vi "Lab Panel V5.26.vi"() -> ()   [LabVIEW 2017] (continued)
                          tunnel: w859 -> [_ _ w868]
                          tunnel: w858 -> [w866 w867 _]
                          tunnel: [w866 w867 w868] -> w857
                          frame "CHART TEST", Default {
                          }
                          frame "CYCLE TEST" {
                          }
                          frame "T-RISE TEST" {
                          }
                        }
                        n587 = local read "TDMS LAB01-2"() -> (w865:refnum<k34>)
                        n588 = Build Array("STOPPED") -> (w862:string[])
                        n589 = Build Array(w857) -> (w856:dbl[])
                        n590 = TDMS Write(0:w865, 5:"TEST RESULT", 7:w862, 9:w856) -> (4:w854:refnum<k34>, 15:w855:errorcluster)  [unwired: 2 in, 2 out]
                        n591 = TDMS Close(8:w855, 11:w854) -> (0:w853:errorcluster)  [unwired: 1 out]
                      }
                      frame #1 {
                        n592 = local read "DISP LAB01-2"() -> (w872:T4)
                        n593 = stacked-sequence {
                          tunnel: "LAB01-2" -> [w874 w876]
                          frame #0 {
                            n594 = call "sub vi - defrag tdms v1.vi"("panel id"=w874) -> ("error out"=w873:errorcluster)  [unwired: 10 in]
                            n595 = local write "data file error"(w873) -> ()
                          }
                          frame #1 {
                            n596 = call "Save data file (stop) v3.vi"("panel id"=w876) -> ("network file save error"=w875:errorcluster)  [unwired: 9 in, 1 out]
                            n597 = local write "RESULT LAB01-2"(FALSE) -> ()
                            n598 = local write "data file error"(w875) -> ()
                          }
                        }
                        n599 = Bundle(cluster=w872, "STATUS"="STOP") -> (w870:T4)  [unwired: 2 in]
                        n600 = local write "DISP LAB01-2"(w870) -> ()
                      }
                    }
                  }
                  frame True {
                    n601 = local read "SIG LAB01-2"() -> (w879:T2)
                    n602 = stacked-sequence {
                      seq-local: [w890 _] -> [_ w894]
                      tunnel: w888 -> [_ w904]
                      tunnel: w887 -> [_ w903]
                      tunnel: w886 -> [_ w902]
                      tunnel: w885 -> [_ w901]
                      tunnel: w884 -> [_ w900]
                      tunnel: [_ w899] -> w883
                      tunnel: w882 -> [_ w898]
                      tunnel: w881 -> [_ w897]
                      tunnel: w880 -> [_ w896]
                      tunnel: w879 -> [w889 w895]
                      tunnel: w878 -> [_ w893]
                      frame #0 {
                        n603 = Unbundle(w889) -> ("AMPS"=w892:dbl)  [unwired: 4 out]
                        n604 = call "Check For Amps on v1.vi"("ID"="LAB01-2", "amps"=w892) -> ("amps"=w890:bool)  [unwired: 9 in]
                      }
                      frame #1 {
                        n605 = case shown="True" w894 {
                          tunnel: w904 -> [_ w917]
                          tunnel: w903 -> [_ w916]
                          tunnel: w902 -> [_ w915]
                          tunnel: w901 -> [_ w914]
                          tunnel: w900 -> [_ w913]
                          tunnel: [errorcluster {"status"=FALSE, "code"=0, "source"=""} ("error out") w912] -> w899
                          tunnel: w898 -> [_ w911]
                          tunnel: w897 -> [_ w910]
                          tunnel: w896 -> [_ w909]
                          tunnel: w895 -> [_ w908]
                          tunnel: w893 -> [_ w907]
                          frame False {
                            w905 = FALSE
                            n606 = local write "RUN LAB01-2"(w905) -> ()
                            n607 = local write "run lab01-2"(w905) -> ()
                          }
                          frame True {
                            n608 = stacked-sequence {
                              seq-local: [w918 _ _ _ _] -> [_ w942 _ _ _]
                              tunnel: w917 -> [w923 _ _ _ _]
                              tunnel: w916 -> [w920 _ _ _ _]
                              tunnel: w915 -> [w933 _ _ _ _]
                              tunnel: w914 -> [w926 _ _ _ _]
                              tunnel: w913 -> [w921 _ _ _ _]
                              tunnel: [_ w937 _ _ _] -> w912
                              tunnel: w911 -> [_ _ _ w964 _]
                              tunnel: w910 -> [_ _ _ w963 _]
                              tunnel: w909 -> [_ _ _ w962 _]
                              tunnel: w908 -> [_ _ _ _ _]
                              tunnel: w907 -> [_ _ _ _ w977]
                              frame #0 {
                                w919 = "\\"
                                n609 = local read "SET LAB01-2"() -> (w928:T5)
                                n610 = case shown="\"CYCLE TEST\"" w933 {
                                tunnel: ["L01-2-CHART TEST-" "L01-2-CYCLE TEST-" "L01-2-T-RISE TEST-"] -> w929
                                frame "CHART TEST", Default {
                                }
                                frame "CYCLE TEST" {
                                }
                                frame "T-RISE TEST" {
                                }
                                }
                                n611 = Unbundle(w928) -> ("DESCRIPTION"=w927:string)  [unwired: 4 out]
                                n612 = Concatenate Strings(w923, "\\", w921, w919, w920, w919) -> (w930:string)
                                n613 = String To Path(string=w930) -> (path=w932:path)
                                n614 = Concatenate Strings(w930, w929, w927, "-", w926, ".tdms") -> (w918:string)
                                n615 = Create Folder(path (use dialog)=w932) -> (error out=w931:errorcluster)  [unwired: 2 in, 2 out]
                                n616 = call <vilib>:"Clear Errors.vi"("error in (no error)"=w931) -> ()  [unwired: 5 in, 2 out]
                                n617 = global write "Global 1.vi" "LAB01-2 FILE"(w918) -> ()
                              }
                              frame #1 {
                                (unwired) FALSE
                                n618 = String To Path(string=w942) -> (path=w938:path)
                                n619 = TDMS Open(6:FALSE, 10:T21."create or replace" ("operation (0:open)"), 11:w938) -> (0:w937:errorcluster, 3:→"TDMS LAB01-2":refnum<k34>)  [unwired: 4 in]
                              }
                              frame #2 {
                                n620 = local read "SET LAB01-2"() -> (w948:T5)
                                n621 = local read "TDMS LAB01-2"() -> (w959:refnum<k34>)
                                n622 = Build Array("Testers Name", "Description", "Set Test Cycles", "T-Rise minutes", "T-Rise Deg C") -> (w949:string[])
                                n623 = Unbundle(w948) -> ("NAME"=w947:string, "DESCRIPTION"=w946:string, "CYCLES"=w945:dbl, "T-RISE mins"=w944:dbl, "T-RISE deg C"=w943:dbl)
                                n624 = Number To Decimal String(number=w945) -> (decimal integer string=w958:string)  [unwired: 1 in]
                                n625 = Number To Decimal String(number=w944) -> (decimal integer string=w957:string)  [unwired: 1 in]
                                n626 = Number To Decimal String(number=w943) -> (decimal integer string=w956:string)  [unwired: 1 in]
                                n627 = Build Array(w947, w946, w958, w957, w956) -> (w955:string[])
                                n628 = TDMS Set Properties(5:w955, 7:w949, 11:w959) -> ()  [unwired: 3 in, 4 out]
                              }
                              frame #3 {
                                n629 = local read "DISP LAB01-2"() -> (w961:T4)
                                n630 = Concatenate Strings("LAB01-2  ", w964) -> (w965:string)
                                n631 = Two Button Dialog(message=w965, 1:w962, 2:w963) -> (T button?=w967:bool)
                                n632 = case shown="True" w967 {
                                tunnel: w961 -> [w974 w975]
                                tunnel: [w974 w975] -> w971
                                tunnel: [w973 w976] -> w970
                                tunnel: [w972 w976] -> w969
                                frame False {
                                n633 = Unbundle(w974) -> ("CYCLE"=w973:dbl, "MINS"=w972:dbl)  [unwired: 1 out]
                                }
                                frame True {
                                w976 = 0.0
                                }
                                }
                                n634 = Bundle(cluster=w971, "CYCLE"=w970, "MINS"=w969, "STATUS"="RUN") -> (w960:T4)
                                n635 = local write "DISP LAB01-2"(w960) -> ()
                              }
                              frame #4 {
                                n636 = local read "TEMP START LAB01-2"() -> (w979:cluster{"TL":dbl, "TN":dbl})
                                n637 = Bundle(cluster=w979, "TL"=w977, "TN"=w977) -> (w978:cluster{"TL":dbl, "TN":dbl})
                                n638 = local write "TEMP START LAB01-2"(w978) -> ()
                              }
                            }
                          }
                        }
                      }
                    }
                  }
                }
              }
              event "RUN LAB02-1": Value Change {
                n639 = event-data() -> ("NewVal"=w985:bool)  [unwired: 1 in, 5 out]
                n640 = local read "SIG LAB02-1"() -> (w981:T2)
                n641 = case shown="True" w985 {
                  tunnel: w991 -> [_ w1029]
                  tunnel: w990 -> [_ w1028]
                  tunnel: w988 -> [w993 w1027]
                  tunnel: w989 -> [_ w1026]
                  tunnel: w987 -> [_ w1025]
                  tunnel: [w992 w1024] -> w986
                  tunnel: w984 -> [_ w1023]
                  tunnel: w983 -> [_ w1022]
                  tunnel: w982 -> [_ w1021]
                  tunnel: w981 -> [_ w1020]
                  tunnel: w980 -> [_ w1019]
                  frame False {
                    # "stop test"
                    n642 = stacked-sequence {
                      tunnel: w993 -> [w1002 _]
                      tunnel: [w994 _] -> w992
                      frame #0 {
                        n643 = local read "DISP LAB02-1"() -> (w1001:T4)
                        n644 = Unbundle(w1001) -> ("CYCLE"=w999:dbl, "MINS"=w1000:dbl)  [unwired: 1 out]
                        n645 = case shown="\"CYCLE TEST\"" w1002 {
                          tunnel: w1000 -> [_ _ w1009]
                          tunnel: w999 -> [w1007 w1008 _]
                          tunnel: [w1007 w1008 w1009] -> w998
                          frame "CHART TEST", Default {
                          }
                          frame "CYCLE TEST" {
                          }
                          frame "T-RISE TEST" {
                          }
                        }
                        n646 = local read "TDMS LAB02-1"() -> (w1006:refnum<k34>)
                        n647 = Build Array("STOPPED") -> (w1003:string[])
                        n648 = Build Array(w998) -> (w997:dbl[])
                        n649 = TDMS Write(0:w1006, 5:"TEST RESULT", 7:w1003, 9:w997) -> (4:w995:refnum<k34>, 15:w996:errorcluster)  [unwired: 2 in, 2 out]
                        n650 = TDMS Close(8:w996, 11:w995) -> (0:w994:errorcluster)  [unwired: 1 out]
                      }
                      frame #1 {
                        n651 = local read "DISP LAB02-1"() -> (w1013:T4)
                        n652 = stacked-sequence {
                          tunnel: "LAB02-1" -> [w1015 w1017]
                          frame #0 {
                            n653 = call "sub vi - defrag tdms v1.vi"("panel id"=w1015) -> ("error out"=w1014:errorcluster)  [unwired: 10 in]
                            n654 = local write "data file error"(w1014) -> ()
                          }
                          frame #1 {
                            n655 = local write "RESULT LAB02-1"(FALSE) -> ()
                            n656 = call "Save data file (stop) v3.vi"("panel id"=w1017) -> ("network file save error"=w1016:errorcluster)  [unwired: 9 in, 1 out]
                            n657 = local write "data file error"(w1016) -> ()
                          }
                        }
                        n658 = Bundle(cluster=w1013, "STATUS"="STOP") -> (w1011:T4)  [unwired: 2 in]
                        n659 = local write "DISP LAB02-1"(w1011) -> ()
                      }
                    }
                  }
                  frame True {
                    n660 = stacked-sequence {
                      seq-local: [w1031 _] -> [_ w1035]
                      tunnel: w1029 -> [_ w1045]
                      tunnel: w1028 -> [_ w1044]
                      tunnel: w1027 -> [_ w1043]
                      tunnel: w1026 -> [_ w1042]
                      tunnel: w1025 -> [_ w1041]
                      tunnel: [_ w1040] -> w1024
                      tunnel: w1023 -> [_ w1039]
                      tunnel: w1022 -> [_ w1038]
                      tunnel: w1021 -> [_ w1037]
                      tunnel: w1020 -> [w1030 w1036]
                      tunnel: w1019 -> [_ w1034]
                      frame #0 {
                        n661 = Unbundle(w1030) -> ("AMPS"=w1033:dbl)  [unwired: 4 out]
                        n662 = call "Check For Amps on v1.vi"("ID"="LAB02-1", "amps"=w1033) -> ("amps"=w1031:bool)  [unwired: 9 in]
                      }
                      frame #1 {
                        n663 = case shown="True" w1035 {
                          tunnel: w1045 -> [_ w1058]
                          tunnel: w1044 -> [_ w1057]
                          tunnel: w1043 -> [_ w1056]
                          tunnel: w1042 -> [_ w1055]
                          tunnel: w1041 -> [_ w1054]
                          tunnel: [errorcluster {"status"=FALSE, "code"=0, "source"=""} ("error out") w1053] -> w1040
                          tunnel: w1039 -> [_ w1052]
                          tunnel: w1038 -> [_ w1051]
                          tunnel: w1037 -> [_ w1050]
                          tunnel: w1036 -> [_ w1049]
                          tunnel: w1034 -> [_ w1048]
                          frame False {
                            w1047 = FALSE
                            n664 = local write "RUN LAB02-1"(w1047) -> ()
                            n665 = local write "run lab02-1"(w1047) -> ()
                          }
                          frame True {
                            n666 = stacked-sequence {
                              seq-local: [w1059 _ _ _ _] -> [_ w1083 _ _ _]
                              tunnel: w1058 -> [w1064 _ _ _ _]
                              tunnel: w1057 -> [w1061 _ _ _ _]
                              tunnel: w1056 -> [w1074 _ _ _ _]
                              tunnel: w1055 -> [w1067 _ _ _ _]
                              tunnel: w1054 -> [w1062 _ _ _ _]
                              tunnel: [_ w1078 _ _ _] -> w1053
                              tunnel: w1052 -> [_ _ _ w1104 _]
                              tunnel: w1051 -> [_ _ _ w1103 _]
                              tunnel: w1050 -> [_ _ _ w1102 _]
                              tunnel: w1049 -> [_ _ _ _ _]
                              tunnel: w1048 -> [_ _ _ _ w1118]
                              frame #0 {
                                w1060 = "\\"
                                n667 = local read "SET LAB02-1"() -> (w1069:T5)
                                n668 = case shown="\"CYCLE TEST\"" w1074 {
                                tunnel: ["L02-1-CHART TEST-" "L02-1-CYCLE TEST-" "L02-1-T-RISE TEST-"] -> w1070
                                frame "CHART TEST", Default {
                                }
                                frame "CYCLE TEST" {
                                }
                                frame "T-RISE TEST" {
                                }
                                }
                                n669 = Unbundle(w1069) -> ("DESCRIPTION"=w1068:string)  [unwired: 4 out]
                                n670 = Concatenate Strings(w1064, "\\", w1062, w1060, w1061, w1060) -> (w1071:string)
                                n671 = String To Path(string=w1071) -> (path=w1073:path)
                                n672 = Concatenate Strings(w1071, w1070, w1068, "-", w1067, ".tdms") -> (w1059:string)
                                n673 = Create Folder(path (use dialog)=w1073) -> (error out=w1072:errorcluster)  [unwired: 2 in, 2 out]
                                n674 = global write "Global 1.vi" "LAB02-1 FILE"(w1059) -> ()
                                n675 = call <vilib>:"Clear Errors.vi"("error in (no error)"=w1072) -> ()  [unwired: 5 in, 2 out]
                              }
                              frame #1 {
                                (unwired) FALSE
                                n676 = String To Path(string=w1083) -> (path=w1079:path)
                                n677 = TDMS Open(6:FALSE, 10:T21."create or replace" ("operation (0:open)"), 11:w1079) -> (0:w1078:errorcluster, 3:→"TDMS LAB02-1":refnum<k34>)  [unwired: 4 in]
                              }
                              frame #2 {
                                n678 = local read "SET LAB02-1"() -> (w1089:T5)
                                n679 = local read "TDMS LAB02-1"() -> (w1100:refnum<k34>)
                                n680 = Build Array("Testers Name", "Description", "Set Test Cycles", "T-Rise minutes", "T-Rise Deg C") -> (w1090:string[])
                                n681 = Unbundle(w1089) -> ("NAME"=w1088:string, "DESCRIPTION"=w1087:string, "CYCLES"=w1086:dbl, "T-RISE mins"=w1085:dbl, "T-RISE deg C"=w1084:dbl)
                                n682 = Number To Decimal String(number=w1086) -> (decimal integer string=w1099:string)  [unwired: 1 in]
                                n683 = Number To Decimal String(number=w1085) -> (decimal integer string=w1098:string)  [unwired: 1 in]
                                n684 = Number To Decimal String(number=w1084) -> (decimal integer string=w1097:string)  [unwired: 1 in]
                                n685 = Build Array(w1088, w1087, w1099, w1098, w1097) -> (w1096:string[])
                                n686 = TDMS Set Properties(5:w1096, 7:w1090, 11:w1100) -> ()  [unwired: 3 in, 4 out]
                              }
                              frame #3 {
                                n687 = local read "DISP LAB02-1"() -> (w1105:T4)
                                n688 = Concatenate Strings("LAB02-1  ", w1104) -> (w1106:string)
                                n689 = Two Button Dialog(message=w1106, 1:w1102, 2:w1103) -> (T button?=w1108:bool)
                                n690 = case shown="True" w1108 {
                                tunnel: w1105 -> [w1115 w1116]
                                tunnel: [w1115 w1116] -> w1112
                                tunnel: [w1114 w1117] -> w1111
                                tunnel: [w1113 w1117] -> w1110
                                frame False {
                                n691 = Unbundle(w1115) -> ("CYCLE"=w1114:dbl, "MINS"=w1113:dbl)  [unwired: 1 out]
                                }
                                frame True {
                                w1117 = 0.0
                                }
                                }
                                n692 = Bundle(cluster=w1112, "CYCLE"=w1111, "MINS"=w1110, "STATUS"="RUN") -> (w1101:T4)
                                n693 = local write "DISP LAB02-1"(w1101) -> ()
                              }
                              frame #4 {
                                n694 = local read "TEMP START LAB02-1"() -> (w1120:cluster{"TL":dbl, "TN":dbl})
                                n695 = Bundle(cluster=w1120, "TL"=w1118, "TN"=w1118) -> (w1119:cluster{"TL":dbl, "TN":dbl})
                                n696 = local write "TEMP START LAB02-1"(w1119) -> ()
                              }
                            }
                          }
                        }
                      }
                    }
                  }
                }
                n697 = local write "run lab02-1"(w985) -> ()
              }
              event "RUN LAB02-2": Value Change {
                n698 = event-data() -> ("NewVal"=w1125:bool)  [unwired: 1 in, 5 out]
                n699 = local write "run lab02-2"(w1125) -> ()
                n700 = case shown="True" w1125 {
                  tunnel: w1131 -> [_ w1169]
                  tunnel: w1130 -> [_ w1168]
                  tunnel: w1128 -> [w1133 w1167]
                  tunnel: w1129 -> [_ w1166]
                  tunnel: w1127 -> [_ w1165]
                  tunnel: [w1132 w1164] -> w1126
                  tunnel: w1124 -> [_ w1163]
                  tunnel: w1123 -> [_ w1162]
                  tunnel: w1122 -> [_ w1161]
                  tunnel: w1121 -> [_ w1159]
                  frame False {
                    # "stop test"
                    n701 = stacked-sequence {
                      tunnel: w1133 -> [w1142 _]
                      tunnel: [w1134 _] -> w1132
                      frame #0 {
                        n702 = local read "DISP LAB02-2"() -> (w1141:T4)
                        n703 = Unbundle(w1141) -> ("CYCLE"=w1139:dbl, "MINS"=w1140:dbl)  [unwired: 1 out]
                        n704 = case shown="\"CYCLE TEST\"" w1142 {
                          tunnel: w1140 -> [_ _ w1149]
                          tunnel: w1139 -> [w1147 w1148 _]
                          tunnel: [w1147 w1148 w1149] -> w1138
                          frame "CHART TEST", Default {
                          }
                          frame "CYCLE TEST" {
                          }
                          frame "T-RISE TEST" {
                          }
                        }
                        n705 = local read "TDMS LAB02-2"() -> (w1146:refnum<k34>)
                        n706 = Build Array("STOPPED") -> (w1143:string[])
                        n707 = Build Array(w1138) -> (w1137:dbl[])
                        n708 = TDMS Write(0:w1146, 5:"TEST RESULT", 7:w1143, 9:w1137) -> (4:w1135:refnum<k34>, 15:w1136:errorcluster)  [unwired: 2 in, 2 out]
                        n709 = TDMS Close(8:w1136, 11:w1135) -> (0:w1134:errorcluster)  [unwired: 1 out]
                      }
                      frame #1 {
                        n710 = local read "DISP LAB02-2"() -> (w1153:T4)
                        n711 = stacked-sequence {
                          tunnel: "LAB02-2" -> [w1155 w1157]
                          frame #0 {
                            n712 = call "sub vi - defrag tdms v1.vi"("panel id"=w1155) -> ("error out"=w1154:errorcluster)  [unwired: 10 in]
                            n713 = local write "data file error"(w1154) -> ()
                          }
                          frame #1 {
                            n714 = call "Save data file (stop) v3.vi"("panel id"=w1157) -> ("network file save error"=w1156:errorcluster)  [unwired: 9 in, 1 out]
                            n715 = local write "RESULT LAB02-2"(FALSE) -> ()
                            n716 = local write "data file error"(w1156) -> ()
                          }
                        }
                        n717 = Bundle(cluster=w1153, "STATUS"="STOP") -> (w1151:T4)  [unwired: 2 in]
                        n718 = local write "DISP LAB02-2"(w1151) -> ()
                      }
                    }
                  }
                  frame True {
                    n719 = local read "SIG LAB02-2"() -> (w1160:T2)
                    n720 = stacked-sequence {
                      seq-local: [w1171 _] -> [_ w1175]
                      tunnel: w1169 -> [_ w1185]
                      tunnel: w1168 -> [_ w1184]
                      tunnel: w1167 -> [_ w1183]
                      tunnel: w1166 -> [_ w1182]
                      tunnel: w1165 -> [_ w1181]
                      tunnel: [_ w1180] -> w1164
                      tunnel: w1163 -> [_ w1179]
                      tunnel: w1162 -> [_ w1178]
                      tunnel: w1161 -> [_ w1177]
                      tunnel: w1160 -> [w1170 w1176]
                      tunnel: w1159 -> [_ w1174]
                      frame #0 {
                        n721 = Unbundle(w1170) -> ("AMPS"=w1173:dbl)  [unwired: 4 out]
                        n722 = call "Check For Amps on v1.vi"("ID"="LAB02-2", "amps"=w1173) -> ("amps"=w1171:bool)  [unwired: 9 in]
                      }
                      frame #1 {
                        n723 = case shown="True" w1175 {
                          tunnel: w1185 -> [_ w1198]
                          tunnel: w1184 -> [_ w1197]
                          tunnel: w1183 -> [_ w1196]
                          tunnel: w1182 -> [_ w1195]
                          tunnel: w1181 -> [_ w1194]
                          tunnel: [errorcluster {"status"=FALSE, "code"=0, "source"=""} ("error out") w1193] -> w1180
                          tunnel: w1179 -> [_ w1192]
                          tunnel: w1178 -> [_ w1191]
                          tunnel: w1177 -> [_ w1190]
                          tunnel: w1176 -> [_ w1189]
                          tunnel: w1174 -> [_ w1188]
                          frame False {
                            w1186 = FALSE
                            n724 = local write "RUN LAB02-2"(w1186) -> ()
                            n725 = local write "run lab02-2"(w1186) -> ()
                          }
                          frame True {
                            n726 = stacked-sequence {
                              seq-local: [w1199 _ _ _ _] -> [_ w1223 _ _ _]
                              tunnel: w1198 -> [w1204 _ _ _ _]
                              tunnel: w1197 -> [w1201 _ _ _ _]
                              tunnel: w1196 -> [w1214 _ _ _ _]
                              tunnel: w1195 -> [w1207 _ _ _ _]
                              tunnel: w1194 -> [w1202 _ _ _ _]
                              tunnel: [_ w1218 _ _ _] -> w1193
                              tunnel: w1192 -> [_ _ _ w1244 _]
                              tunnel: w1191 -> [_ _ _ w1243 _]
                              tunnel: w1190 -> [_ _ _ w1242 _]
                              tunnel: w1189 -> [_ _ _ _ _]
                              tunnel: w1188 -> [_ _ _ _ w1258]
                              frame #0 {
                                w1200 = "\\"
                                n727 = local read "SET LAB02-2"() -> (w1209:T5)
                                n728 = case shown="\"CYCLE TEST\"" w1214 {
                                tunnel: ["L02-2-CHART TEST-" "L02-2-CYCLE TEST-" "L02-2-T-RISE TEST-"] -> w1210
                                frame "CHART TEST", Default {
                                }
                                frame "CYCLE TEST" {
                                }
                                frame "T-RISE TEST" {
                                }
                                }
                                n729 = Unbundle(w1209) -> ("DESCRIPTION"=w1208:string)  [unwired: 4 out]
                                n730 = Concatenate Strings(w1204, "\\", w1202, w1200, w1201, w1200) -> (w1211:string)
                                n731 = String To Path(string=w1211) -> (path=w1213:path)
                                n732 = Concatenate Strings(w1211, w1210, w1208, "-", w1207, ".tdms") -> (w1199:string)
                                n733 = Create Folder(path (use dialog)=w1213) -> (error out=w1212:errorcluster)  [unwired: 2 in, 2 out]
                                n734 = global write "Global 1.vi" "LAB02-2 FILE"(w1199) -> ()
                                n735 = call <vilib>:"Clear Errors.vi"("error in (no error)"=w1212) -> ()  [unwired: 5 in, 2 out]
                              }
                              frame #1 {
                                (unwired) FALSE
                                n736 = String To Path(string=w1223) -> (path=w1219:path)
                                n737 = TDMS Open(6:FALSE, 10:T21."create or replace" ("operation (0:open)"), 11:w1219) -> (0:w1218:errorcluster, 3:→"TDMS LAB02-2":refnum<k34>)  [unwired: 4 in]
                              }
                              frame #2 {
                                n738 = local read "SET LAB02-2"() -> (w1229:T5)
                                n739 = local read "TDMS LAB02-2"() -> (w1240:refnum<k34>)
                                n740 = Build Array("Testers Name", "Description", "Set Test Cycles", "T-Rise minutes", "T-Rise Deg C") -> (w1230:string[])
                                n741 = Unbundle(w1229) -> ("NAME"=w1228:string, "DESCRIPTION"=w1227:string, "CYCLES"=w1226:dbl, "T-RISE mins"=w1225:dbl, "T-RISE deg C"=w1224:dbl)
                                n742 = Number To Decimal String(number=w1226) -> (decimal integer string=w1239:string)  [unwired: 1 in]
                                n743 = Number To Decimal String(number=w1225) -> (decimal integer string=w1238:string)  [unwired: 1 in]
                                n744 = Number To Decimal String(number=w1224) -> (decimal integer string=w1237:string)  [unwired: 1 in]
                                n745 = Build Array(w1228, w1227, w1239, w1238, w1237) -> (w1236:string[])
                                n746 = TDMS Set Properties(5:w1236, 7:w1230, 11:w1240) -> ()  [unwired: 3 in, 4 out]
                              }
                              frame #3 {
                                n747 = local read "DISP LAB02-2"() -> (w1245:T4)
                                n748 = Concatenate Strings("LAB02-2  ", w1244) -> (w1246:string)
                                n749 = Two Button Dialog(message=w1246, 1:w1242, 2:w1243) -> (T button?=w1248:bool)
                                n750 = case shown="True" w1248 {
                                tunnel: w1245 -> [w1255 w1256]
                                tunnel: [w1255 w1256] -> w1252
                                tunnel: [w1254 w1257] -> w1251
                                tunnel: [w1253 w1257] -> w1250
                                frame False {
                                n751 = Unbundle(w1255) -> ("CYCLE"=w1254:dbl, "MINS"=w1253:dbl)  [unwired: 1 out]
                                }
                                frame True {
                                w1257 = 0.0
                                }
                                }
                                n752 = Bundle(cluster=w1252, "CYCLE"=w1251, "MINS"=w1250, "STATUS"="RUN") -> (w1241:T4)
                                n753 = local write "DISP LAB02-2"(w1241) -> ()
                              }
                              frame #4 {
                                n754 = local read "TEMP START LAB02-2"() -> (w1260:cluster{"TL":dbl, "TN":dbl})
                                n755 = Bundle(cluster=w1260, "TL"=w1258, "TN"=w1258) -> (w1259:cluster{"TL":dbl, "TN":dbl})
                                n756 = local write "TEMP START LAB02-2"(w1259) -> ()
                              }
                            }
                          }
                        }
                      }
                    }
                  }
                }
              }
              event "RUN LAB03-1": Value Change {
                n757 = event-data() -> ("NewVal"=w1265:bool)  [unwired: 1 in, 5 out]
                n758 = local write "run lab03-1"(w1265) -> ()
                n759 = case shown="True" w1265 {
                  tunnel: w1271 -> [_ w1309]
                  tunnel: w1270 -> [_ w1308]
                  tunnel: w1268 -> [w1273 w1307]
                  tunnel: w1269 -> [_ w1306]
                  tunnel: w1267 -> [_ w1305]
                  tunnel: [w1272 w1304] -> w1266
                  tunnel: w1264 -> [_ w1303]
                  tunnel: w1263 -> [_ w1302]
                  tunnel: w1262 -> [_ w1301]
                  tunnel: w1261 -> [_ w1299]
                  frame False {
                    # "stop test"
                    n760 = stacked-sequence {
                      tunnel: w1273 -> [w1282 _]
                      tunnel: [w1274 _] -> w1272
                      frame #0 {
                        n761 = local read "DISP LAB03-1"() -> (w1281:T4)
                        n762 = Unbundle(w1281) -> ("CYCLE"=w1279:dbl, "MINS"=w1280:dbl)  [unwired: 1 out]
                        n763 = case shown="\"CYCLE TEST\"" w1282 {
                          tunnel: w1280 -> [_ _ w1289]
                          tunnel: w1279 -> [w1287 w1288 _]
                          tunnel: [w1287 w1288 w1289] -> w1278
                          frame "CHART TEST", Default {
                          }
                          frame "CYCLE TEST" {
                          }
                          frame "T-RISE TEST" {
                          }
                        }
                        n764 = local read "TDMS LAB03-1"() -> (w1286:refnum<k34>)
                        n765 = Build Array("STOPPED") -> (w1283:string[])
                        n766 = Build Array(w1278) -> (w1277:dbl[])
                        n767 = TDMS Write(0:w1286, 5:"TEST RESULT", 7:w1283, 9:w1277) -> (4:w1275:refnum<k34>, 15:w1276:errorcluster)  [unwired: 2 in, 2 out]
                        n768 = TDMS Close(8:w1276, 11:w1275) -> (0:w1274:errorcluster)  [unwired: 1 out]
                      }
                      frame #1 {
                        n769 = local read "DISP LAB03-1"() -> (w1293:T4)
                        n770 = stacked-sequence {
                          tunnel: "LAB03-1" -> [w1295 w1297]
                          frame #0 {
                            n771 = call "sub vi - defrag tdms v1.vi"("panel id"=w1295) -> ("error out"=w1294:errorcluster)  [unwired: 10 in]
                            n772 = local write "data file error"(w1294) -> ()
                          }
                          frame #1 {
                            n773 = call "Save data file (stop) v3.vi"("panel id"=w1297) -> ("network file save error"=w1296:errorcluster)  [unwired: 9 in, 1 out]
                            n774 = local write "RESULT LAB03-1"(FALSE) -> ()
                            n775 = local write "data file error"(w1296) -> ()
                          }
                        }
                        n776 = Bundle(cluster=w1293, "STATUS"="STOP") -> (w1291:T4)  [unwired: 2 in]
                        n777 = local write "DISP LAB03-1"(w1291) -> ()
                      }
                    }
                  }
                  frame True {
                    n778 = local read "SIG LAB03-1"() -> (w1300:T2)
                    n779 = stacked-sequence {
                      seq-local: [w1311 _] -> [_ w1315]
                      tunnel: w1309 -> [_ w1325]
                      tunnel: w1308 -> [_ w1324]
                      tunnel: w1307 -> [_ w1323]
                      tunnel: w1306 -> [_ w1322]
                      tunnel: w1305 -> [_ w1321]
                      tunnel: [_ w1320] -> w1304
                      tunnel: w1303 -> [_ w1319]
                      tunnel: w1302 -> [_ w1318]
                      tunnel: w1301 -> [_ w1317]
                      tunnel: w1300 -> [w1310 w1316]
                      tunnel: w1299 -> [_ w1314]
                      frame #0 {
                        n780 = Unbundle(w1310) -> ("AMPS"=w1313:dbl)  [unwired: 4 out]
                        n781 = call "Check For Amps on v1.vi"("ID"="LAB03-1", "amps"=w1313) -> ("amps"=w1311:bool)  [unwired: 9 in]
                      }
                      frame #1 {
                        n782 = case shown="True" w1315 {
                          tunnel: w1325 -> [_ w1338]
                          tunnel: w1324 -> [_ w1337]
                          tunnel: w1323 -> [_ w1336]
                          tunnel: w1322 -> [_ w1335]
                          tunnel: w1321 -> [_ w1334]
                          tunnel: [errorcluster {"status"=FALSE, "code"=0, "source"=""} ("error out") w1333] -> w1320
                          tunnel: w1319 -> [_ w1332]
                          tunnel: w1318 -> [_ w1331]
                          tunnel: w1317 -> [_ w1330]
                          tunnel: w1316 -> [_ w1329]
                          tunnel: w1314 -> [_ w1328]
                          frame False {
                            w1326 = FALSE
                            n783 = local write "RUN LAB03-1"(w1326) -> ()
                            n784 = local write "run lab03-1"(w1326) -> ()
                          }
                          frame True {
                            n785 = stacked-sequence {
                              seq-local: [w1339 _ _ _ _] -> [_ w1363 _ _ _]
                              tunnel: w1338 -> [w1344 _ _ _ _]
                              tunnel: w1337 -> [w1341 _ _ _ _]
                              tunnel: w1336 -> [w1354 _ _ _ _]
                              tunnel: w1335 -> [w1347 _ _ _ _]
                              tunnel: w1334 -> [w1342 _ _ _ _]
                              tunnel: [_ w1358 _ _ _] -> w1333
                              tunnel: w1332 -> [_ _ _ w1383 _]
                              tunnel: w1331 -> [_ _ _ w1382 _]
                              tunnel: w1330 -> [_ _ _ w1381 _]
                              tunnel: w1329 -> [_ _ _ _ _]
                              tunnel: w1328 -> [_ _ _ _ w1398]
                              frame #0 {
                                w1340 = "\\"
                                n786 = local read "SET LAB03-1"() -> (w1349:T5)
                                n787 = case shown="\"T-RISE TEST\"" w1354 {
                                tunnel: ["L03-1-CHART TEST-" "L03-1-CYCLE TEST-" "L03-1-T-RISE TEST-"] -> w1350
                                frame "CHART TEST", Default {
                                }
                                frame "CYCLE TEST" {
                                }
                                frame "T-RISE TEST" {
                                }
                                }
                                n788 = Unbundle(w1349) -> ("DESCRIPTION"=w1348:string)  [unwired: 4 out]
                                n789 = Concatenate Strings(w1344, "\\", w1342, w1340, w1341, w1340) -> (w1351:string)
                                n790 = String To Path(string=w1351) -> (path=w1353:path)
                                n791 = Concatenate Strings(w1351, w1350, w1348, "-", w1347, ".tdms") -> (w1339:string)
                                n792 = Create Folder(path (use dialog)=w1353) -> (error out=w1352:errorcluster)  [unwired: 2 in, 2 out]
                                n793 = global write "Global 1.vi" "LAB03-1 FILE"(w1339) -> ()
                                n794 = call <vilib>:"Clear Errors.vi"("error in (no error)"=w1352) -> ()  [unwired: 5 in, 2 out]
                              }
                              frame #1 {
                                (unwired) FALSE
                                n795 = String To Path(string=w1363) -> (path=w1359:path)
                                n796 = TDMS Open(6:FALSE, 10:T21."create or replace" ("operation (0:open)"), 11:w1359) -> (0:w1358:errorcluster, 3:→"TDMS LAB03-1":refnum<k34>)  [unwired: 4 in]
                              }
                              frame #2 {
                                n797 = local read "SET LAB03-1"() -> (w1369:T5)
                                n798 = local read "TDMS LAB03-1"() -> (w1380:refnum<k34>)
                                n799 = Build Array("Testers Name", "Description", "Set Test Cycles", "T-Rise minutes", "T-Rise Deg C") -> (w1370:string[])
                                n800 = Unbundle(w1369) -> ("NAME"=w1368:string, "DESCRIPTION"=w1367:string, "CYCLES"=w1366:dbl, "T-RISE mins"=w1365:dbl, "T-RISE deg C"=w1364:dbl)
                                n801 = Number To Decimal String(number=w1366) -> (decimal integer string=w1379:string)  [unwired: 1 in]
                                n802 = Number To Decimal String(number=w1365) -> (decimal integer string=w1378:string)  [unwired: 1 in]
                                n803 = Number To Decimal String(number=w1364) -> (decimal integer string=w1377:string)  [unwired: 1 in]
                                n804 = Build Array(w1368, w1367, w1379, w1378, w1377) -> (w1376:string[])
                                n805 = TDMS Set Properties(5:w1376, 7:w1370, 11:w1380) -> ()  [unwired: 3 in, 4 out]
                              }
                              frame #3 {
                                n806 = local read "DISP LAB03-1"() -> (w1385:T4)
                                n807 = Concatenate Strings("LAB03-1  ", w1383) -> (w1386:string)
                                n808 = Two Button Dialog(message=w1386, 1:w1381, 2:w1382) -> (T button?=w1388:bool)
                                n809 = case shown="True" w1388 {
                                tunnel: w1385 -> [w1395 w1396]
                                tunnel: [w1395 w1396] -> w1392
                                tunnel: [w1394 w1397] -> w1391
                                tunnel: [w1393 w1397] -> w1390
                                frame False {
                                n810 = Unbundle(w1395) -> ("CYCLE"=w1394:dbl, "MINS"=w1393:dbl)  [unwired: 1 out]
                                }
                                frame True {
                                w1397 = 0.0
                                }
                                }
                                n811 = Bundle(cluster=w1392, "CYCLE"=w1391, "MINS"=w1390, "STATUS"="RUN") -> (w1384:T4)
                                n812 = local write "DISP LAB03-1"(w1384) -> ()
                              }
                              frame #4 {
                                n813 = local read "TEMP START LAB03-1"() -> (w1400:cluster{"TL":dbl, "TN":dbl})
                                n814 = Bundle(cluster=w1400, "TL"=w1398, "TN"=w1398) -> (w1399:cluster{"TL":dbl, "TN":dbl})
                                n815 = local write "TEMP START LAB03-1"(w1399) -> ()
                              }
                            }
                          }
                        }
                      }
                    }
                  }
                }
              }
              event "RUN LAB03-2": Value Change {
                n816 = event-data() -> ("NewVal"=w1405:bool)  [unwired: 1 in, 5 out]
                n817 = local write "run lab03-2"(w1405) -> ()
                n818 = case shown="True" w1405 {
                  tunnel: w1411 -> [_ w1449]
                  tunnel: w1410 -> [_ w1448]
                  tunnel: w1408 -> [w1413 w1447]
                  tunnel: w1409 -> [_ w1446]
                  tunnel: w1407 -> [_ w1445]
                  tunnel: [w1412 w1444] -> w1406
                  tunnel: w1404 -> [_ w1443]
                  tunnel: w1403 -> [_ w1442]
                  tunnel: w1402 -> [_ w1441]
                  tunnel: w1401 -> [_ w1439]
                  frame False {
                    # "stop test"
                    n819 = stacked-sequence {
                      tunnel: w1413 -> [w1422 _]
                      tunnel: [w1414 _] -> w1412
                      frame #0 {
                        n820 = local read "DISP LAB03-2"() -> (w1421:T4)
                        n821 = Unbundle(w1421) -> ("CYCLE"=w1419:dbl, "MINS"=w1420:dbl)  [unwired: 1 out]
                        n822 = case shown="\"CYCLE TEST\"" w1422 {
                          tunnel: w1420 -> [_ _ w1429]
                          tunnel: w1419 -> [w1427 w1428 _]
                          tunnel: [w1427 w1428 w1429] -> w1418
                          frame "CHART TEST", Default {
                          }
                          frame "CYCLE TEST" {
                          }
                          frame "T-RISE TEST" {
                          }
                        }
                        n823 = local read "TDMS LAB03-2"() -> (w1426:refnum<k34>)
                        n824 = Build Array("STOPPED") -> (w1423:string[])
                        n825 = Build Array(w1418) -> (w1417:dbl[])
                        n826 = TDMS Write(0:w1426, 5:"TEST RESULT", 7:w1423, 9:w1417) -> (4:w1415:refnum<k34>, 15:w1416:errorcluster)  [unwired: 2 in, 2 out]
                        n827 = TDMS Close(8:w1416, 11:w1415) -> (0:w1414:errorcluster)  [unwired: 1 out]
                      }
                      frame #1 {
                        n828 = local read "DISP LAB03-2"() -> (w1433:T4)
                        n829 = stacked-sequence {
                          tunnel: "LAB03-2" -> [w1435 w1437]
                          frame #0 {
                            n830 = call "sub vi - defrag tdms v1.vi"("panel id"=w1435) -> ("error out"=w1434:errorcluster)  [unwired: 10 in]
                            n831 = local write "data file error"(w1434) -> ()
                          }
                          frame #1 {
                            n832 = call "Save data file (stop) v3.vi"("panel id"=w1437) -> ("network file save error"=w1436:errorcluster)  [unwired: 9 in, 1 out]
                            n833 = local write "RESULT LAB03-2"(FALSE) -> ()
                            n834 = local write "data file error"(w1436) -> ()
                          }
                        }
                        n835 = Bundle(cluster=w1433, "STATUS"="STOP") -> (w1431:T4)  [unwired: 2 in]
                        n836 = local write "DISP LAB03-2"(w1431) -> ()
                      }
                    }
                  }
                  frame True {
                    n837 = local read "SIG LAB03-2"() -> (w1440:T2)
                    n838 = stacked-sequence {
                      seq-local: [w1451 _] -> [_ w1455]
                      tunnel: w1449 -> [_ w1465]
                      tunnel: w1448 -> [_ w1464]
                      tunnel: w1447 -> [_ w1463]
                      tunnel: w1446 -> [_ w1462]
                      tunnel: w1445 -> [_ w1461]
                      tunnel: [_ w1460] -> w1444
                      tunnel: w1443 -> [_ w1459]
                      tunnel: w1442 -> [_ w1458]
                      tunnel: w1441 -> [_ w1457]
                      tunnel: w1440 -> [w1450 w1456]
                      tunnel: w1439 -> [_ w1454]
                      frame #0 {
                        n839 = Unbundle(w1450) -> ("AMPS"=w1453:dbl)  [unwired: 4 out]
                        n840 = call "Check For Amps on v1.vi"("ID"="LAB03-2", "amps"=w1453) -> ("amps"=w1451:bool)  [unwired: 9 in]
                      }
                      frame #1 {
                        n841 = case shown="True" w1455 {
                          tunnel: w1465 -> [_ w1478]
                          tunnel: w1464 -> [_ w1477]
                          tunnel: w1463 -> [_ w1476]
                          tunnel: w1462 -> [_ w1475]
                          tunnel: w1461 -> [_ w1474]
                          tunnel: [errorcluster {"status"=FALSE, "code"=0, "source"=""} ("error out") w1473] -> w1460
                          tunnel: w1459 -> [_ w1472]
                          tunnel: w1458 -> [_ w1471]
                          tunnel: w1457 -> [_ w1470]
                          tunnel: w1456 -> [_ w1469]
                          tunnel: w1454 -> [_ w1468]
                          frame False {
                            w1466 = FALSE
                            n842 = local write "RUN LAB03-2"(w1466) -> ()
                            n843 = local write "run lab03-2"(w1466) -> ()
                          }
                          frame True {
                            n844 = stacked-sequence {
                              seq-local: [w1479 _ _ _ _] -> [_ w1503 _ _ _]
                              tunnel: w1478 -> [w1484 _ _ _ _]
                              tunnel: w1477 -> [w1481 _ _ _ _]
                              tunnel: w1476 -> [w1494 _ _ _ _]
                              tunnel: w1475 -> [w1487 _ _ _ _]
                              tunnel: w1474 -> [w1482 _ _ _ _]
                              tunnel: [_ w1498 _ _ _] -> w1473
                              tunnel: w1472 -> [_ _ _ w1524 _]
                              tunnel: w1471 -> [_ _ _ w1523 _]
                              tunnel: w1470 -> [_ _ _ w1522 _]
                              tunnel: w1469 -> [_ _ _ _ _]
                              tunnel: w1468 -> [_ _ _ _ w1538]
                              frame #0 {
                                w1480 = "\\"
                                n845 = local read "SET LAB03-2"() -> (w1489:T5)
                                n846 = case shown="\"T-RISE TEST\"" w1494 {
                                tunnel: ["L03-2-CHART TEST-" "L03-2-CYCLE TEST-" "L03-2-T-RISE TEST-"] -> w1490
                                frame "CHART TEST", Default {
                                }
                                frame "CYCLE TEST" {
                                }
                                frame "T-RISE TEST" {
                                }
                                }
                                n847 = Unbundle(w1489) -> ("DESCRIPTION"=w1488:string)  [unwired: 4 out]
                                n848 = Concatenate Strings(w1484, "\\", w1482, w1480, w1481, w1480) -> (w1491:string)
                                n849 = String To Path(string=w1491) -> (path=w1493:path)
                                n850 = Concatenate Strings(w1491, w1490, w1488, "-", w1487, ".tdms") -> (w1479:string)
                                n851 = Create Folder(path (use dialog)=w1493) -> (error out=w1492:errorcluster)  [unwired: 2 in, 2 out]
                                n852 = global write "Global 1.vi" "LAB03-2 FILE"(w1479) -> ()
                                n853 = call <vilib>:"Clear Errors.vi"("error in (no error)"=w1492) -> ()  [unwired: 5 in, 2 out]
                              }
                              frame #1 {
                                (unwired) FALSE
                                n854 = String To Path(string=w1503) -> (path=w1499:path)
